vi "GitLog.vi"(6 "skip":i32 min=0 step=1, 8 "error in (no error)":errorcluster, 9 "Directory":path=path "", 10 "Number":i32=1 min=1 step=1, 11 "Git exec":string="git") -> (0 "error out":errorcluster, 1 "Directory out":path, 2 "Commit Info":T1[](array[typedef]), 3 "Git exec out":string="git")   [LabVIEW 2013]
uses:
  GitCommitCluster/CommitCluster.ctl
  GitCmd.vi
  <vilib>/dlg_ctls.llb/Space Constant.vi
  GitUtils/PathtoDirPath.vi
  <vilib>/Platform/system.llb/System Exec.vi
  <vilib>/Utility/error.llb/Error Cluster From Error Code.vi
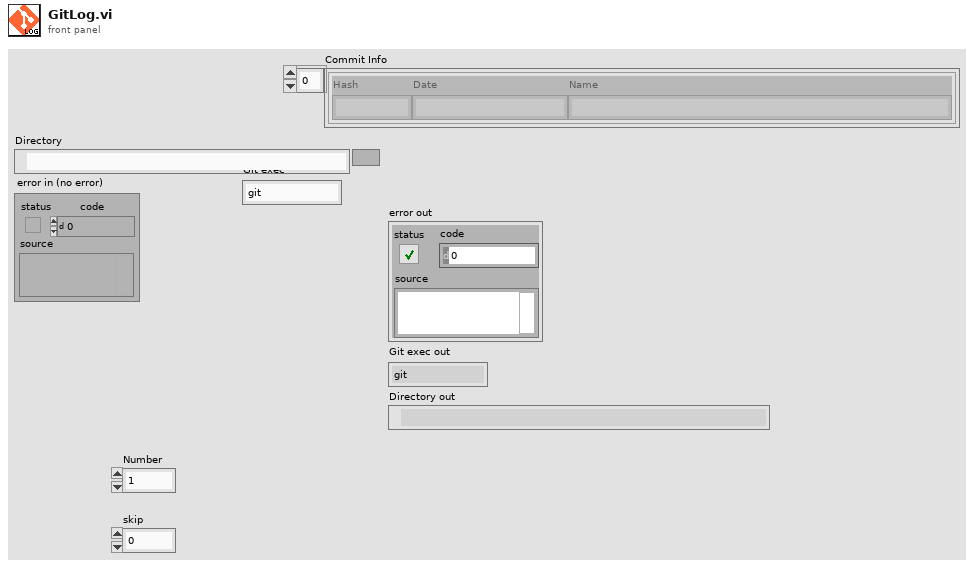
[diagram p1: front panel]
types:
  T1 = typedef "CommitCluster.ctl" = cluster{"Hash":string, "Date":string, "Name":string}
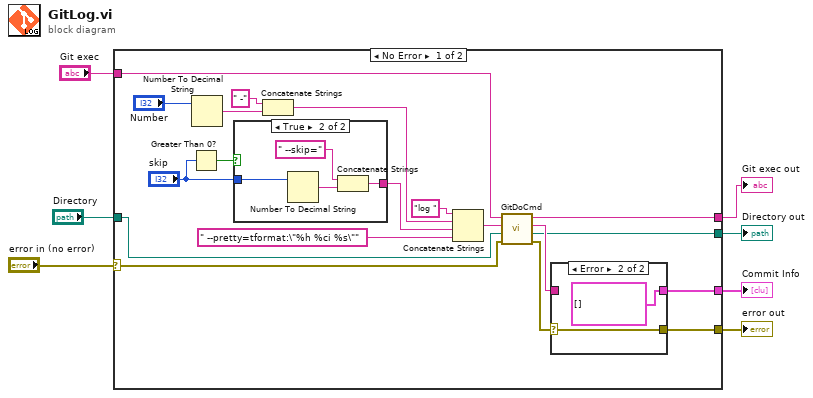
[diagram p0: block diagram]
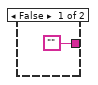
[diagram p2: hidden frame]
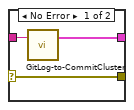
[diagram p3: hidden frame]
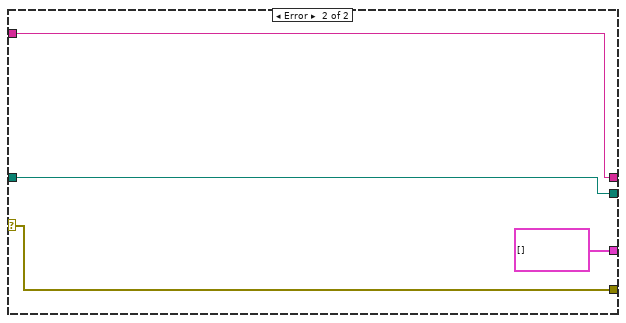
[diagram p4: hidden frame]
diagram:
  n1 = case shown="No Error" "error in (no error)" {
    selector: "error in (no error)" -> [w15 w40]
    tunnel: "Git exec" -> [w12 w38]
    tunnel: "Directory" -> [w8 w37]
    tunnel: [w17 T1[] [] ("Array")] -> w4
    tunnel: [w16 w40] -> w5
    tunnel: [w11 w38] -> w2
    tunnel: [w9 w37] -> w1
    frame No Error {
      n2 = Greater Than 0?(x="skip") -> (x > 0?=w21:bool)
      n3 = Number To Decimal String(number="Number") -> (decimal integer string=w24:string)  [unwired: 1 in]
      n4 = case shown="True" w21 {
        tunnel: "skip" -> [_ w31]
        tunnel: ["" w28] -> w19
        frame False {
        }
        frame True {
          n5 = Number To Decimal String(number=w31) -> (decimal integer string=w30:string)  [unwired: 1 in]
          n6 = Concatenate Strings(" --skip=" ("string"), w30) -> (w28:string)
        }
      }
      n7 = Concatenate Strings(" -" ("string"), w24) -> (w22:string)
      n8 = Concatenate Strings("log " ("string"), w22, w19, " --pretty=tformat:\"%h %ci %s\"" ("string")) -> (w13:string)
      n9 = call "GitDoCmd.vi"("error in (no error)"=w15, "Working Path"=w8, "Git command"=w13, "Git exec"=w12) -> ("error out"=w14:errorcluster, "Working Path out"=w9:path, "Returned stdout"=w10:string, "Git exec out"=w11:string)  [unwired: 3 in]
      n10 = case shown="Error" w14 {
        selector: w14 -> [w32 w35]
        tunnel: w10 -> [w34 _]
        tunnel: [w33 T1[] [] ("Array")] -> w17
        tunnel: [w32 w35] -> w16
        frame No Error {
          n11 = call "GitLog-to-CommitCluster.vi"("Git Log In"=w34) -> ("Array"=w33:T1[])  [unwired: 2 in]
        }
        frame Error {
        }
      }
    }
    frame Error {
    }
  }
  "error out" <- w5
  "Git exec out" <- w2
  "Directory out" <- w1
  "Commit Info" <- w4
